vi "ReadNumber.vi"(8 "error in (no error)":errorcluster, 11 "SimpleDevice in":refnum<class "SimpleDevice.lvclass">) -> (0 "error out":errorcluster, 2 "Number":dbl, 3 "SimpleDevice out":refnum<class "SimpleDevice.lvclass">)   [LabVIEW 2021, in "SimpleDevice.lvlib" / "SimpleDevice.lvclass"]
uses:
  SimpleDevice.lvclass
  SimpleDevice.lvclass/SimpleDevice.ctl
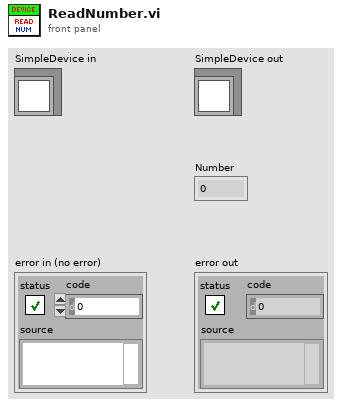
[diagram p1: front panel]
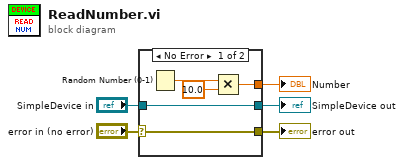
[diagram p0: block diagram]
diagram:
  n1 = case shown="No Error" "error in (no error)" {
    selector: "error in (no error)" -> [w9 w12]
    tunnel: [w9 w12] -> w4
    tunnel: [w10 w11] -> w2
    tunnel: "SimpleDevice in" -> [w10 w11]
    tunnel: [w7 _] -> w1
    frame No Error {
      n2 = Random Number (0-1)() -> (number: 0 to 1=w8:dbl)
      n3 = Multiply(x=w8, y=10.0) -> (x*y=w7:dbl)
    }
    frame Error {
    }
  }
  "error out" <- w4
  "SimpleDevice out" <- w2
  "Number" <- w1
